vi "Sorted Particle Report.vi"(2 "Area Size Limit":dbl, 3 "Particle Count Limit":dbl=inf, 4 "Pixel Measurements":T1[](array[typedef])=[35, 4, 5, 6, 7] items=["Center of Mass X", "Center of Mass Y", "First Pixel X", "First Pixel Y", "Bounding Rect Left", "Bounding Rect Top", "Bounding Rect Right", "Bounding Rect Bottom", "Max Feret Diameter Start X", "Max Feret Diameter Start Y", "Max Feret Diameter End X", "Max Feret Diameter End Y", "Max Horiz. Segment Length Left", "Max Horiz. Segment Length Right", "Max Horiz. Segment Length Row", "-", "Bounding Rect Width", "Bounding Rect Height", "Bounding Rect Diagonal", "Perimeter", "Convex Hull Perimeter", "Holes' Perimeter", "Max Feret Diameter", "Equivalent Ellipse Major Axis", "Equivalent Ellipse Minor Axis", "Equivalent Ellipse Minor Axis (Feret)", "Equivalent Rect Long Side", "Equivalent Rect Short Side", "Equivalent Rect Diagonal", "Equivalent Rect Short Side (Feret)", "Average Horiz. Segment Length", "Average Vert. Segment Length", "Hydraulic Radius", "Waddel Disk Diameter", "-", "Area", "Holes' Area", "Particle & Holes' Area", "Convex Hull Area", "Image Area", "-", "Number of Holes", "Number of Horiz. Segments", "Number of Vert. Segments", "-", "Orientation", "Max Feret Diameter Orientation", "-", "% Area/Image Area", "% Area/(Particle & Holes' Area)", "Ratio of Equivalent Ellipse Axes", "Ratio of Equivalent Rect Sides", "-", "Elongation Factor", "Compactness Factor", "Heywood Circularity Factor", "Type Factor", "-", "Sum X", "Sum Y", "Sum XX", "Sum XY", "Sum YY", "Sum XXX", "Sum XXY", "Sum XYY", "Sum YYY", "-", "Moment of Inertia XX", "Moment of Inertia XY", "Moment of Inertia YY", "Moment of Inertia XXX", "Moment of Inertia XXY", "Moment of Inertia XYY", "Moment of Inertia YYY", "Norm. Moment of Inertia XX", "Norm. Moment of Inertia XY", "Norm. Moment of Inertia YY", "Norm. Moment of Inertia XXX", "Norm. Moment of Inertia XXY", "Norm. Moment of Inertia XYY", "Norm. Moment of Inertia YYY", "Hu Moment 1", "Hu Moment 2", "Hu Moment 3", "Hu Moment 4", "Hu Moment 5", "Hu Moment 6", "Hu Moment 7"], 5 "Image in":T2) -> (0 "Sorted Data":dbl[][](array[numeric]), 1 "Particles":i32)   [LabVIEW 2025]
doc: "Returns the requested measurements of a binary image sorted by the first parameter (often size), and limiting the rows in the 2D array by count or size. Pass infinity to count to avoid a limit. Pass zero to size to avoid a limit."
uses:
  <vilib>/vision/Image Controls.llb/IMAQ Image.ctl
  <vilib>/vision/NI_Vision_Development_Module.lvlib
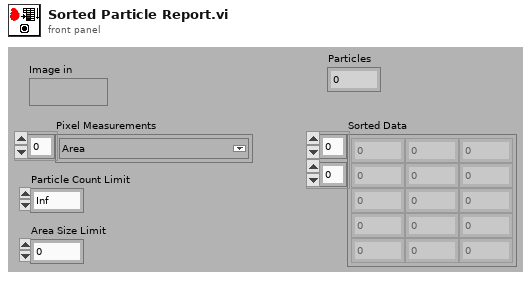
[diagram p1: front panel]
types:
  T1 = typedef "Particle Parameters" = i32
  T2 = typedef "IMAQ Image.ctl" = refnum<image>
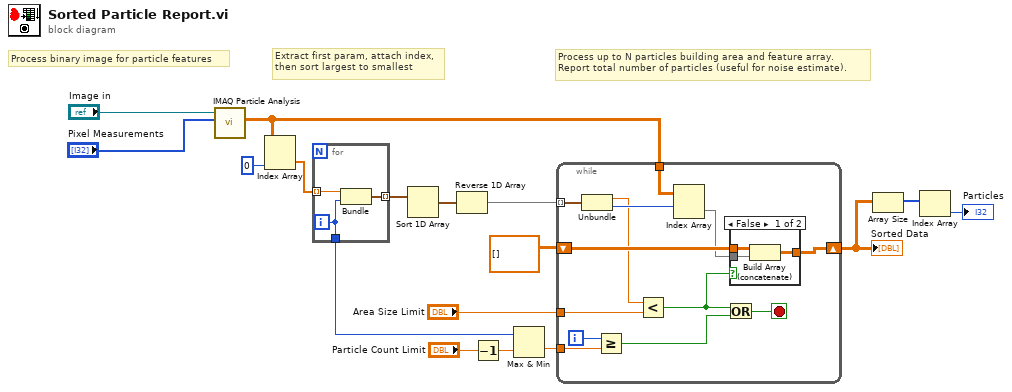
[diagram p0: block diagram]
diagram:
  # "Process up to N particles building area and feature array.\nReport total number of particles (useful for noise estimate)."
  # "Process binary image for particle features"
  # "Extract first param, attach index,\nthen sort largest to smallest"
  n1 = call "IMAQ Particle Analysis"("Pixel Measurements"="Pixel Measurements", "Image"="Image in") -> ("Particle Measurements (Pixels)"=w11:dbl[][])  [unwired: 3 in, 6 out]
  n2 = Index Array(array=w11, index (col)=0 ("disabled index (col)")) -> (element=w14:dbl[])  [unwired: 1 in]
  n3 = for {
    tunnel: w14 -> [w20] mode=indexing
    tunnel: [w19] -> w15 mode=indexing
    tunnel: [w18] -> w1
    i -> [w18]
    n4 = Bundle("Numeric"=w20, w18) -> (w19:cluster{"Numeric":dbl, i32})  [unwired: 1 out]
  }
  n5 = Sort 1D Array(array=w15) -> (sorted array=w16:cluster{"Numeric":dbl, i32}[])
  n6 = Reverse 1D Array(array=w16) -> (reversed array=w4:cluster{"Numeric":dbl, i32}[])
  n7 = Decrement(x="Particle Count Limit") -> (x-1=w2:dbl)
  n8 = Max & Min(x=w1, y=w2) -> (min(x,y)=w3:dbl)  [unwired: 1 out]
  n9 = while {
    tunnel: w11 -> [w32]
    tunnel: w4 -> [w31] mode=indexing
    shift-right: [w28] -> w7
    shift-left: dbl[][] [] -> [w30]
    tunnel: w3 -> [w26]
    tunnel: "Area Size Limit" -> [w24]
    i -> [w27]
    stop <- w21 stop-if-true
    n10 = Unbundle(w31) -> ("Numeric"=w25:dbl, w33:i32)
    n11 = Greater Or Equal?(x=w27, y=w26) -> (x >= y?=w22:bool)
    n12 = Less?(x=w25, y=w24) -> (x < y?=w23:bool)
    n13 = Index Array(array=w32, index (row)=w33) -> (element=w29:dbl[])  [unwired: 1 in]
    n14 = Or(x=w23, y=w22) -> (x .or. y?=w21:bool)
    n15 = case shown="False" w23 {
      tunnel: w30 -> [w36 w37]
      tunnel: w29 -> [w35 _]
      tunnel: [w34 w37] -> w28
      frame False {
        n16 = Build Array (concatenate)(w36, w35) -> (w34:dbl[][])
      }
      frame True {
      }
    }
  }
  "Sorted Data" <- w7
  n17 = Array Size(array=w7) -> (size(s)=w6:i32[])
  n18 = Index Array(array=w6) -> (element=→"Particles":i32)  [unwired: 1 in]
